vi "MathCad_Matrix_Get_2D strings.vi"(0 "Worksheet Reference":refnum<k7>, 1 "Mathcad.IMatrixValue Refnum":refnum<k7>, 2 "error out 2":errorcluster) -> (3 "Worksheet Reference Out":refnum<k7>, 4 "Mathcad.IMatrixValue Refnum":refnum<k7>, 5 "Array":string[][](array[string]), 6 "error out":errorcluster)   [LabVIEW 2015]
doc: "Gets the value from the reference retrieved from the getrefnum VI."
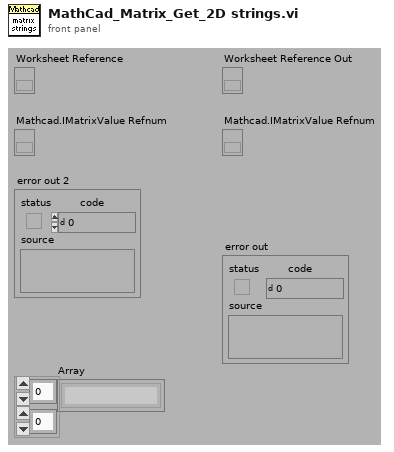
[diagram p1: front panel]
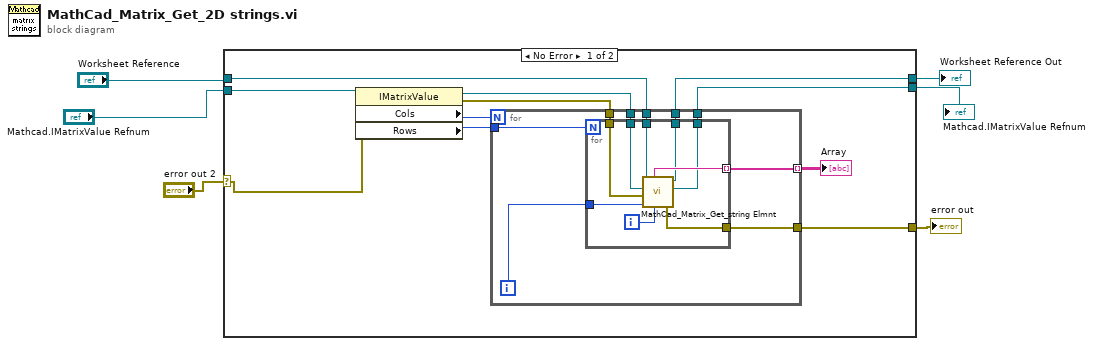
[diagram p0: block diagram]
diagram:
  n1 = case shown="No Error" "error out 2" {
    selector: "error out 2" -> [w17 w38]
    tunnel: "Worksheet Reference" -> [w13 w37]
    tunnel: [w8 w38] -> w5
    tunnel: "Mathcad.IMatrixValue Refnum" -> [w16 w36]
    tunnel: [w10 w37] -> w2
    tunnel: [w9 w36] -> w1
    frame No Error {
      n2 = property class="IMatrixValue"(reference=w16, error in=w17) -> (reference out=w12:refnum<k7>, error out=w11:errorcluster, "Cols"=w15:i32, "Rows"=w14:i32)
      n3 = for {
        N: w15 -> [_]
        tunnel: w14 -> [w26]
        tunnel: w13 -> [w24]
        tunnel: w12 -> [w23]
        tunnel: w11 -> [w22]
        tunnel: [w21] -> w10
        tunnel: [w20] -> w9
        tunnel: [w19] -> w8
        tunnel: [w18] -> w7 mode=indexing
        i -> [w25]
        n4 = for {
          N: w26 -> [_]
          tunnel: w25 -> [w35]
          tunnel: [w33] -> w18 mode=indexing
          tunnel: w24 -> [w32]
          tunnel: w23 -> [w31]
          tunnel: w22 -> [w30]
          tunnel: [w29] -> w21
          tunnel: [w28] -> w20
          tunnel: [w27] -> w19
          i -> [w34]
          n5 = call "MathCad_Matrix_Get_string Elmnt.vi"("row"=w34, "col"=w35, "error in"=w30, "Mathcad.IMatrixValue Refnum"=w31, "Worksheet Reference In"=w32) -> ("error out"=w27:errorcluster, "Mathcad.IMatrixValue Refnum"=w28:refnum<k7>, "Worksheet Reference Out"=w29:refnum<k7>, "string"=w33:string)  [unwired: 1 in]
        }
      }
      "Array" <- w7
    }
    frame Error {
    }
  }
  "Mathcad.IMatrixValue Refnum" <- w1
  "error out" <- w5
  "Worksheet Reference Out" <- w2
